vi "Configure Load to Sequence-Single.vi"(11 "Load to seq config - Single":T1={"Load channel name"="", "Load out"="", "Load sweep values"=[], "Source sweep points"=0, "Load output function"=1007, "Load transient response"=1038, "Load voltage/current gain bandwidth"=0.0, "Load voltage/current compensation frequency"=0.0, "Load voltage/current pole-zero ratio"=0.0, "Load aperture time"=0.0, "Load source delay"=0.0, "Load measure trigger"="", "Load source trigger"=""} {"Load transient response" items=["Slow"=1041, "Normal"=1038, "Fast"=1039, "Custom"=1042]; "Load output function" items=["DC Voltage"=1006, "DC Current"=1007, "Pulse Voltage"=1049, "Pulse Current"=1050]; "Load sweep values" format="%#_13g"}) -> (0 "error out":errorcluster, 3 "instrument handle out":refnum<k15>)   [LabVIEW 2021]
doc: "Configure the load device to sequence mode and trigger load when to start from source and measure trigger."
uses:
  controls/Load to Sequence Config-Single.ctl
  <instrlib>/niDCPower/nidcpower.llb/niDCPower Source Mode.ctl
  <instrlib>/niDCPower/nidcpower.llb/niDCPower Configure Digital Edge Source Trigger With Channels.vi
  <instrlib>/niDCPower/nidcpower.llb/niDCPower Configure Digital Edge Measure Trigger With Channels.vi
panel:
  in  "error in":errorcluster
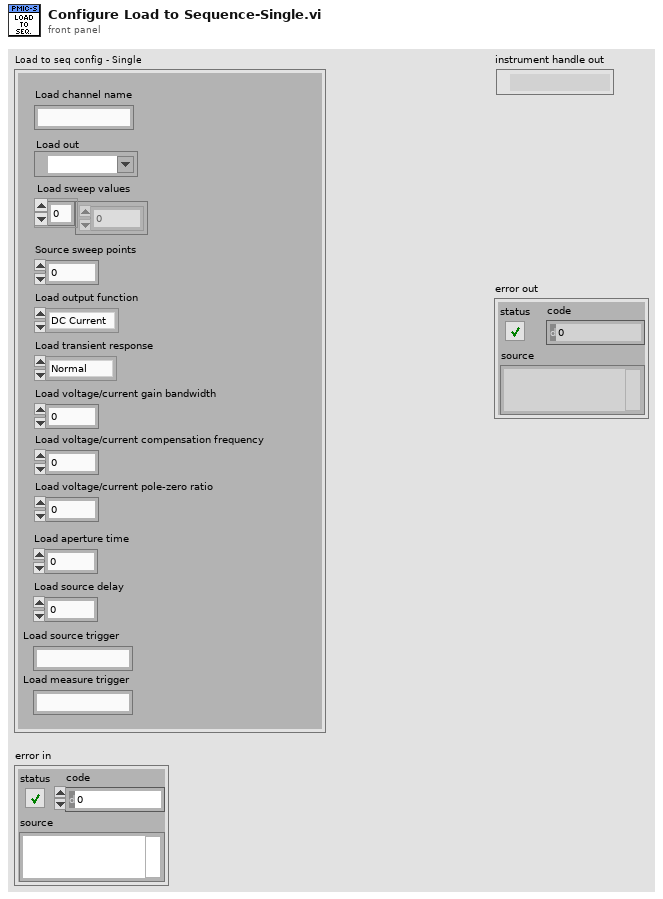
[diagram p1: front panel]
types:
  T1 = typedef "Load to Sequence Config-Single.ctl" = cluster{"Load channel name":string, "Load out":refnum<k15>, "Load sweep values":dbl[], "Source sweep points":i32, "Load output function":i32, "Load transient response":i32, "Load voltage/current gain bandwidth":dbl, "Load voltage/current compensation frequency":dbl, "Load voltage/current pole-zero ratio":dbl, "Load aperture time":dbl, "Load source delay":dbl, "Load measure trigger":string, "Load source trigger":string}
  T2 = typedef "niDCPower Source Mode.ctl" = i32
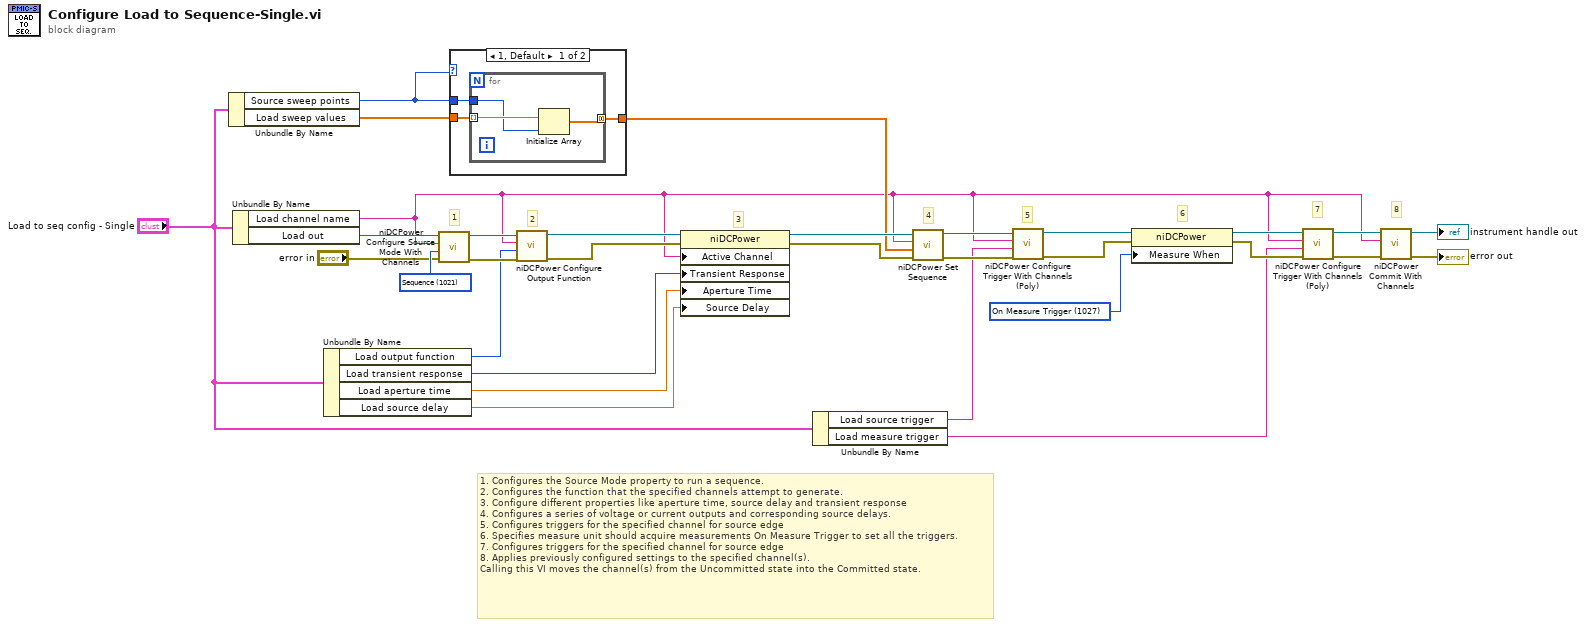
[diagram p0: block diagram]
diagram:
  w14 = 1027 items=["Automatically after Source Complete"=1025, "On Demand"=1026, "On Measure Trigger"=1027] ("Measurement:Advanced:Measure When")
  w30 = T2 1021 items=["Single Point"=1020, "Sequence"=1021] ("source mode")
  # "1. Configures the Source Mode property to run a sequence.\n2. Configures the function that the specified channels attempt to generate.\n3. Configure different properties like aperture time, source delay and transient response\n4. Configures a series of voltage or current outputs and corresponding source delays. \n5. Configures triggers for the specified channel for source edge\n6. Specifies measure unit should acquire measurements On Measure Trigger to set all the triggers.\n7. Configures triggers for the specified channel for source edge\n8. Applies previously configured settings to the specified channel(s).\nCalling this VI moves the channel(s) from the Uncommitted state into the Committed state."
  # "8"
  # "7"
  # "6"
  # "5"
  # "4"
  # "3"
  # "2"
  # "1"
  n1 = Unbundle By Name("Load to seq config - Single") -> ("Source sweep points"=w27:i32, "Load sweep values"=w26:dbl[])
  n2 = Unbundle By Name("Load to seq config - Single") -> ("Load channel name"=w2:string, "Load out"=w31:refnum<k15>)
  n3 = Unbundle By Name("Load to seq config - Single") -> ("Load output function"=w3:i32, "Load transient response"=w22:i32, "Load aperture time"=w23:dbl, "Load source delay"=w4:dbl)
  n4 = call <instrlib>:"niDCPower Configure Source Mode With Channels.vi"("error in (no error)"="error in", "source mode"=w30, "channel name"=w2, "instrument handle"=w31) -> ("error out"=w28:errorcluster, "instrument handle out"=w29:refnum<k15>)  [unwired: 6 in]
  n5 = case shown="1, Default" w27 {
    tunnel: w27 -> [w34 _]
    tunnel: w26 -> [w33 w38]
    tunnel: [w32 w38] -> w19
    frame 1, Default {
      n6 = for {
        tunnel: w34 -> [w35]
        tunnel: w33 -> [w37] mode=indexing
        tunnel: [w36] -> w32 mode=concatenating
        n7 = Initialize Array(w37, w35) -> (w36:dbl[])
      }
    }
    frame 0 {
    }
  }
  n8 = call <instrlib>:"niDCPower Configure Output Function.vi"("error in (no error)"=w28, "output function"=w3, "channel name"=w2, "instrument handle"=w29) -> ("error out"=w24:errorcluster, "instrument handle out"=w25:refnum<k15>)  [unwired: 6 in]
  n9 = property class="niDCPower"(reference=w25, error in=w24, "Active Channel"=w2, "Transient Response"=w22, "Aperture Time"=w23, "Source Delay"=w4) -> (reference out=w21:refnum<k15>, error out=w20:errorcluster)
  n10 = Unbundle By Name("Load to seq config - Single") -> ("Load source trigger"=w6:string, "Load measure trigger"=w7:string)
  n11 = call <instrlib>:"niDCPower Set Sequence.vi"("error in (no error)"=w20, "values"=w19, "channel name"=w2, "instrument handle"=w21) -> ("error out"=w17:errorcluster, "instrument handle out"=w18:refnum<k15>)  [unwired: 6 in]
  n12 = call-poly <instrlib>:"niDCPower Configure Trigger With Channels (Poly).vi"("error in (no error)"=w17, "input terminal"=w6, "channel name"=w2, "instrument handle"=w18) -> ("error out"=w15:errorcluster, "instrument handle out"=w16:refnum<k15>)  [unwired: 6 in]
  n13 = property class="niDCPower"(reference=w16, error in=w15, "Measure When"=w14) -> (reference out=w13:refnum<k15>, error out=w12:errorcluster)
  n14 = call-poly <instrlib>:"niDCPower Configure Trigger With Channels (Poly).vi"("error in (no error)"=w12, "input terminal"=w7, "channel name"=w2, "instrument handle"=w13) -> ("error out"=w10:errorcluster, "instrument handle out"=w11:refnum<k15>)  [unwired: 6 in]
  n15 = call <instrlib>:"niDCPower Commit With Channels.vi"("error in (no error)"=w10, "channel name"=w2, "instrument handle"=w11) -> ("error out"=→"error out":errorcluster, "instrument handle out"=→"instrument handle out":refnum<k15>)  [unwired: 7 in]
